vi "Write IViewable State Queue.vi"(10 "Viewable State Queue":refnum<queue>, 11 "LeakyViewable In":refnum<class "LeakyViewable.lvclass">) -> (3 "LeakyViewable Out":refnum<class "LeakyViewable.lvclass">)   [LabVIEW 2015, in "ViewableDoubles.lvlib" / "LeakyViewable.lvclass"]
uses:
  LeakyViewable.lvclass
  Framework/IViewable/IViewable/IViewable.lvclass
  LeakyViewable.lvclass/LeakyViewable.ctl
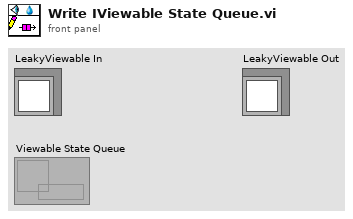
[diagram p1: front panel]
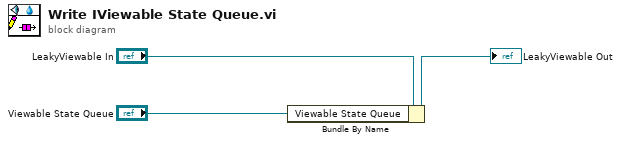
[diagram p0: block diagram]
diagram:
  n1 = Bundle By Name(cluster="LeakyViewable In", "Viewable State Queue"="Viewable State Queue") -> (→"LeakyViewable Out":refnum<class "LeakyViewable.lvclass">)
